vi "get_string_node_terms.vi"(0 "Terms[] In":refnum<vi>[](array[refnum]), 1 "Node Type":T1, 5 "Number of Parameters":i32=1, 11 "error in (no error)":errorcluster) -> (3 "Format Terms Out":refnum<vi>[](array[refnum]), 4 "Terms[]  Out":refnum<vi>[](array[refnum]), 6 "Pick Term":refnum<vi>, 8 "Multiline Term/Enable Term/Concantenate Term":refnum<vi>, 10 "Pick Line Output Term/Disable Term":refnum<vi>, 14 "Bool Output Term":refnum<vi>, 15 "error out":errorcluster)   [LabVIEW 2018]
uses:
  TypeDefinitions/string_node_type.ctl
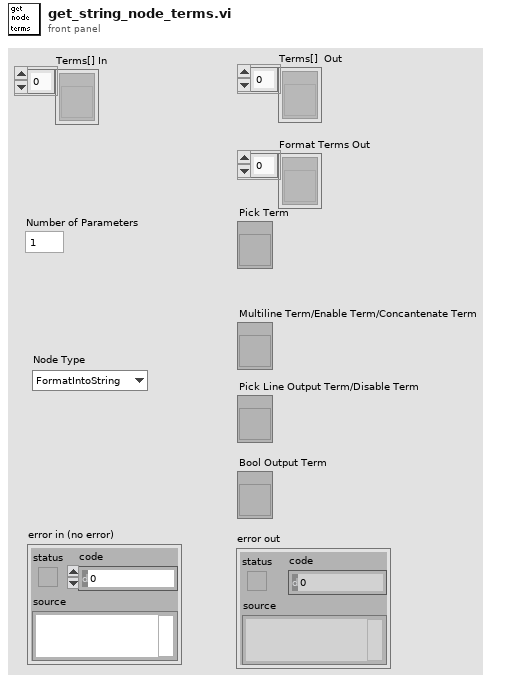
[diagram p1: front panel]
types:
  T1 = typedef "string_node_type.ctl" = enum16{"FormatIntoString", "PickLine", "AppendTrueFalse", "ConcatenateStrings"}
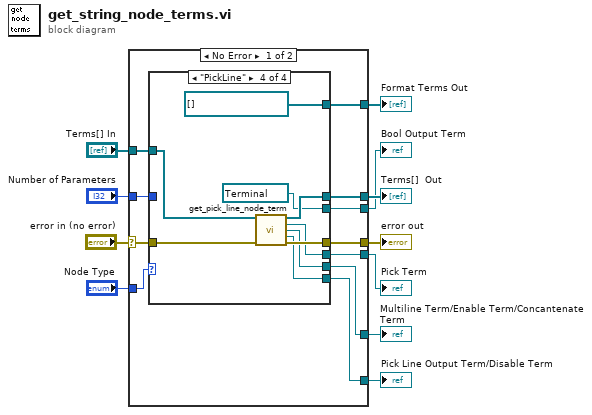
[diagram p0: block diagram]
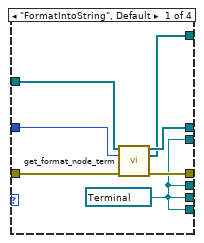
[diagram p2: hidden frame]
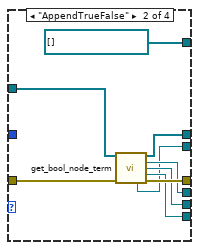
[diagram p3: hidden frame]
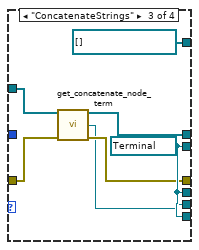
[diagram p4: hidden frame]
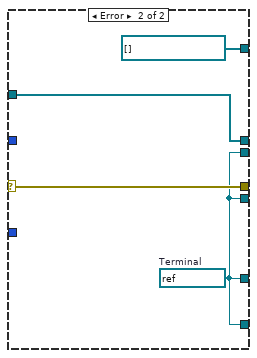
[diagram p5: hidden frame]
diagram:
  n1 = case shown="No Error" "error in (no error)" {
    selector: "error in (no error)" -> [w20 w58]
    tunnel: [w17 w56] -> w11
    tunnel: "Terms[] In" -> [w22 w57]
    tunnel: [w16 w56] -> w9
    tunnel: [w19 w58] -> w7
    tunnel: [w18 w57] -> w6
    tunnel: [w15 w56] -> w5
    tunnel: "Node Type" -> [w21 _]
    tunnel: "Number of Parameters" -> [w14 _]
    tunnel: [w13 refnum<vi>[] [] ("Format Terms Out")] -> w2
    tunnel: [w12 w56] -> w1
    frame No Error {
      n2 = case shown="\"PickLine\"" w21 {
        tunnel: w22 -> [w29 w38 w45 w54]
        tunnel: w20 -> [w27 w37 w44 w53]
        tunnel: [w26 w36 w40 w52] -> w19
        tunnel: [w25 w35 w43 w51] -> w18
        tunnel: [w23 w34 w41 w50] -> w17
        tunnel: [w23 w33 w39 w49] -> w16
        tunnel: [w23 w32 w41 w48] -> w15
        tunnel: w14 -> [w28 _ _ _]
        tunnel: [w24 refnum<vi>[] [] ("Format Terms Out") refnum<vi>[] [] ("Format Terms Out") refnum<vi>[] [] ("Format Terms Out")] -> w13
        tunnel: [w23 w31 w41 refnum<vi> refnum ("Output Term")] -> w12
        frame "FormatIntoString", Default {
          w23 = refnum<vi> refnum ("Pick Term")
          n3 = call "get_format_node_term.vi"("Terms[] In"=w29, "Number of Parameters"=w28, "error in (no error)"=w27) -> ("Terms[]  Out"=w25:refnum<vi>[], "Format Terms Out"=w24:refnum<vi>[], "error out"=w26:errorcluster)  [unwired: 10 out]
        }
        frame "AppendTrueFalse" {
          n4 = call "get_bool_node_term.vi"("Terms[] In"=w38, "error in (no error)"=w37) -> ("Terms[]  Out"=w35:refnum<vi>[], "Pick Term"=w34:refnum<vi>, "Enable Term"=w33:refnum<vi>, "Disable Term"=w32:refnum<vi>, "Output Term"=w31:refnum<vi>, "error out"=w36:errorcluster)  [unwired: 8 out]
        }
        frame "ConcatenateStrings" {
          w41 = refnum<vi> refnum ("Output Term")
          n5 = call "get_concatenate_node_term.vi"("Terms[] In"=w45, "error in (no error)"=w44) -> ("Terms[]  Out"=w43:refnum<vi>[], "Concantenate Term"=w39:refnum<vi>, "error out"=w40:errorcluster)  [unwired: 11 out]
        }
        frame "PickLine" {
          n6 = call "get_pick_line_node_term.vi"("Terms[] In"=w54, "error in (no error)"=w53) -> ("Terms[]  Out"=w51:refnum<vi>[], "Pick Term"=w50:refnum<vi>, "Multiline Term"=w49:refnum<vi>, "Output Ref"=w48:refnum<vi>, "error out"=w52:errorcluster)  [unwired: 9 out]
        }
      }
    }
    frame Error {
      w56 = refnum<vi> refnum  # Terminal
    }
  }
  "Pick Term" <- w11
  "Multiline Term/Enable Term/Concantenate Term" <- w9
  "error out" <- w7
  "Terms[]  Out" <- w6
  "Pick Line Output Term/Disable Term" <- w5
  "Bool Output Term" <- w1
  "Format Terms Out" <- w2
